vi "Import Energies (OSZICAR) from DB.vi"(6 "Reference Energy/atom (pure Crystal) (eV)":dbl=-2.489625, 8 "error in (no error)":errorcluster, 9 "# of Atoms":i32, 10 "OSZICAR ID":string, 11 "connection reference":T3) -> (0 "error out":errorcluster, 1 "Extracted Parameters":T1, 2 "OSZICAR Raw":T2, 3 "connection reference out":T3)   [LabVIEW 2010]
uses:
  <vilib>/addons/database/Connection.llb/Conn ObjectReference.ctl
  <vilib>/addons/database/_DB Variant To Data/Database Variant To Data.xnode
  <vilib>/addons/database/NI_Database_API.lvlib
panel:
  out "Bulk Formation Energies Array (eV)":dbl[](array[numeric])
  out "Ionic Relaxation Energies Array (eV)":dbl[](array[numeric])
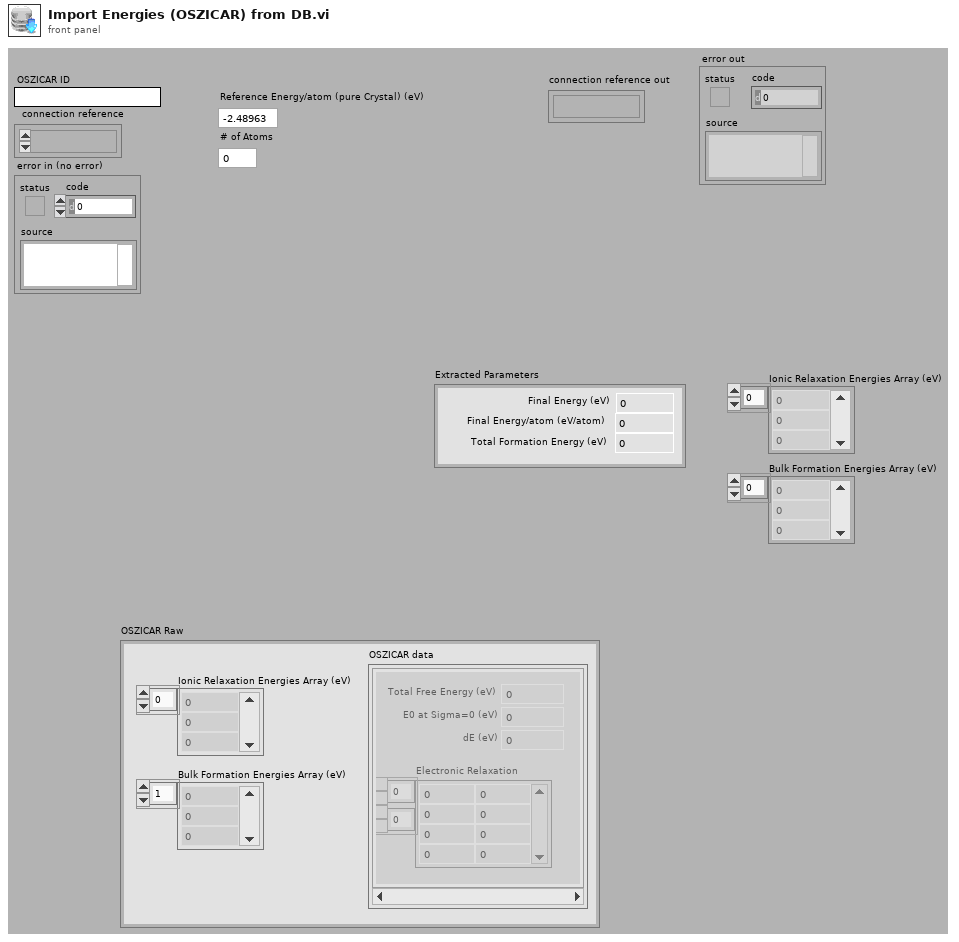
[diagram p1: front panel]
types:
  T1 = cluster{"Final Energy (eV)":dbl, "Final Energy/atom (eV/atom)":dbl, "Total Formation Energy (eV)":dbl}
  T2 = cluster{"OSZICAR data":cluster{"Total Free Energy (eV)":dbl, "E0 at Sigma=0 (eV)":dbl, "dE (eV)":dbl, "Electronic Relaxation":dbl[][]}[], "Ionic Relaxation Energies Array (eV)":dbl[], "Bulk Formation Energies Array (eV)":dbl[]}
  T3 = typedef "NI_Database_API.lvlib/Conn ObjectReference.ctl" = refnum<k1>
  T4 = cluster{"Total Free Energy (eV)":dbl, "E0 at Sigma=0 (eV)":dbl, "dE (eV)":dbl, "Electronic Relaxation":dbl[][]}[]
  T5 = cluster{"OSZICAR data":cluster{"Total Free Energy (eV)":dbl, "E0 at Sigma=0 (eV)":dbl, "dE (eV)":dbl, "Electronic Relaxation":dbl[][]}[], dbl[], dbl[]}
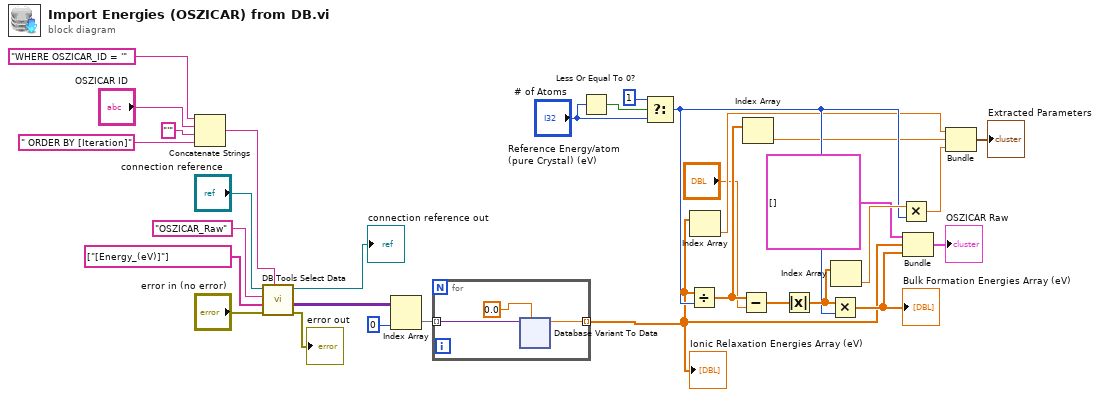
[diagram p0: block diagram]
diagram:
  n1 = Concatenate Strings("WHERE OSZICAR_ID = '", "OSZICAR ID", "'" ("string"), " ORDER BY [Iteration]" ("string")) -> (w24:string)
  n2 = call <vilib>:"DB Tools Select Data.vi"("condition"=w24, "error in (no error)"="error in (no error)", "columns"=string[] ["[Energy_(eV)]"], "table"="OSZICAR_Raw", "connection reference"="connection reference") -> ("error out"=→"error out":errorcluster, "data"=w25:variant[][], "connection reference out"=→"connection reference out":T3)  [unwired: 1 in]
  n3 = Index Array(array=w25, index (col)=0 ("index (row)")) -> (element=w10:variant[])  [unwired: 1 in]
  n4 = for {
    tunnel: w10 -> [w34] mode=indexing
    tunnel: [w33] -> w1 mode=indexing
    n5 = xnode "Database Variant To Data"("database variant"=w34, "type"=0.0) -> ("data"=w33:dbl)  [unwired: 1 in, 1 out]
  }
  "Ionic Relaxation Energies Array (eV)" <- w1
  n6 = Less Or Equal To 0?(x="# of Atoms") -> (x <= 0?=w20:bool)
  n7 = Select(t=1, s=w20, f="# of Atoms") -> (s? t:f=w17:i32)
  n8 = Divide(x=w1, y=w17) -> (x/y=w16:dbl[])
  n9 = Index Array(array=w1) -> (element=w15:dbl)  [unwired: 1 in]
  n10 = Subtract(x=w16, y="Reference Energy/atom (pure Crystal) (eV)") -> (x-y=w22:dbl[])
  n11 = Index Array(array=w16) -> (element=w14:dbl)  [unwired: 1 in]
  n12 = Absolute Value(x=w22) -> (abs(x)=w18:dbl[])
  n13 = Multiply(x=w18, y=w17) -> (x*y=w4:dbl[])
  "Bulk Formation Energies Array (eV)" <- w4
  n14 = Index Array(array=w18) -> (element=w21:dbl)  [unwired: 1 in]
  n15 = Multiply(x=w21, y=w17) -> (x*y=w13:dbl)
  n16 = Bundle("OSZICAR data"=T4 [], w1, w4) -> (→"OSZICAR Raw":T5)  [unwired: 1 in]
  n17 = Bundle("data"=w15, w14, w13) -> (→"Extracted Parameters":cluster{"data":dbl, dbl, dbl})  [unwired: 1 in]
